vi "TAFTraceWindow_SendUiEvent.vi"(7 "UiEventNames":T1, 8 "ErrorIn":errorcluster, 9 "Data":variant, 11 "TAFTraceWindow in":refnum<class "TAFTraceWindow.lvclass">) -> (0 "ErrorOut":errorcluster, 3 "TAFTraceWindow out":refnum<class "TAFTraceWindow.lvclass">)   [LabVIEW 2021, in "TAFTraceWindow.lvclass"]
uses:
  TAFTraceWindow.lvclass
  TAFTraceWindow_UiCallBackEvents.ctl
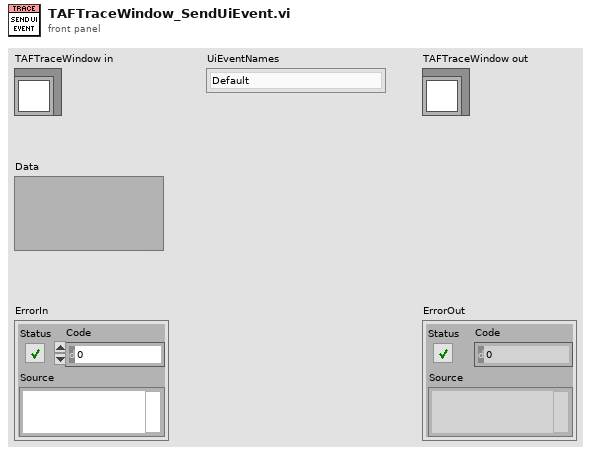
[diagram p1: front panel]
types:
  T1 = typedef "TAFTraceWindow.lvclass/TAFTraceWindow_UiCallBackEvents.ctl" = enum16{"Default", "PersistentDataUpdated"}
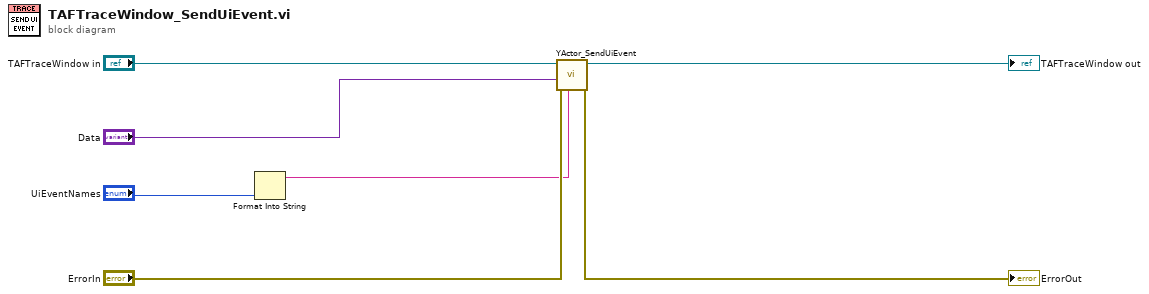
[diagram p0: block diagram]
diagram:
  n1 = Format Into String("UiEventNames") -> (resulting string=w2:string)  [unwired: 3 in, 1 out]
  n2 = call-dynamic "YActor_SendUiEvent.vi"("Event"=w2, "ErrorIn"="ErrorIn", "Data"="Data", "YActorIn"="TAFTraceWindow in") -> ("ErrorOut"=→"ErrorOut":errorcluster, "YActorOut"=→"TAFTraceWindow out":refnum<class "TAFTraceWindow.lvclass">)  [unwired: 6 in]
